vi "Disabled - Split Words from Numbers (SubVI).vi"(7 "Force Reload":bool, 9 "Input Array":string[](array[string]), 11 "File Name":string="Constants.pi") -> (2 "Numeric Array":dbl[](array[numeric]), 3 "Header Array":string[](array[string]))   [LabVIEW 2019]
doc: "Takes a file of the format:\n Line 1: Description\n Line 2: Value\n Line 3: Description\n Line 4: Value\nAnd splits it into a string array of descriptions and a numeric array of constants."
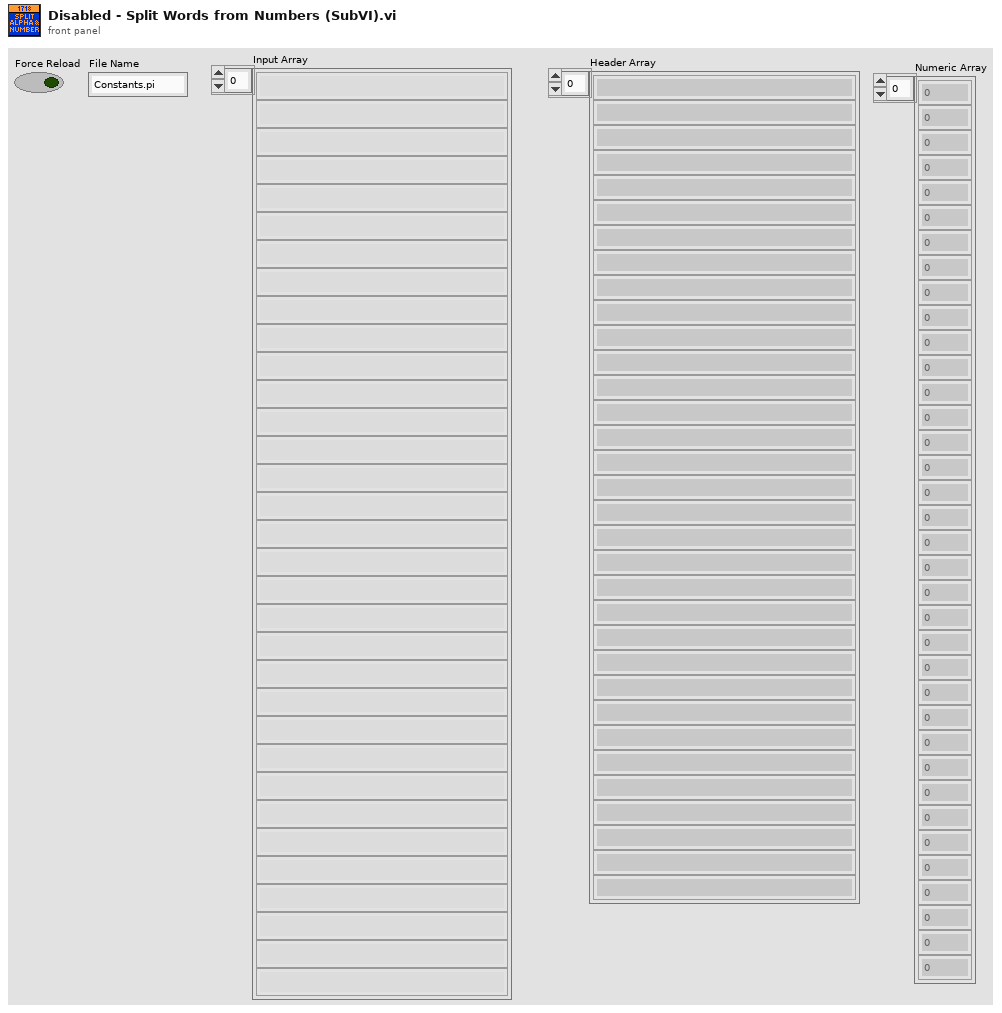
[diagram p1: front panel]
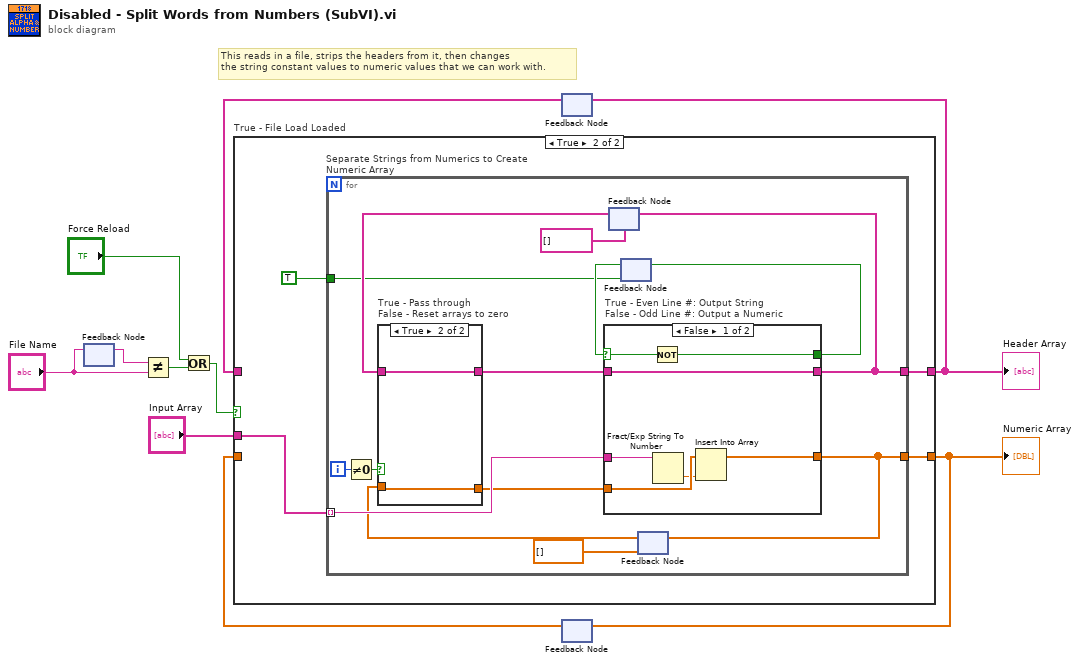
[diagram p0: block diagram]
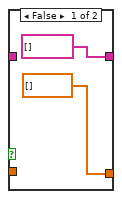
[diagram p3: hidden frame]
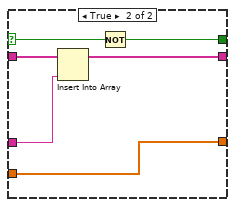
[diagram p4: hidden frame]
diagram:
  # "This reads in a file, strips the headers from it, then changes\nthe string constant values to numeric values that we can work with."
  n1 = feedback-in #1("File Name") -> ()
  n2 = feedback #1() -> (w4:string)  [unwired: 1 in]
  n3 = Not Equal?(x=w4, y="File Name") -> (x != y?=w3:bool)
  n4 = Or(x="Force Reload", y=w3) -> (x .or. y?=w1:bool)
  n5 = feedback #2() -> (w6:string[])  [unwired: 1 in]
  n6 = feedback #3() -> (w7:dbl[])  [unwired: 1 in]
  n7 = case "True - File Load Loaded" shown="True" w1 {
    tunnel: [w12 w16] -> w8
    tunnel: [w11 w15] -> w9
    tunnel: "Input Array" -> [_ w13]
    tunnel: w7 -> [w12 _]
    tunnel: w6 -> [w11 _]
    frame False {
    }
    frame True {
      n8 = for "Separate Strings from Numerics to Create Numeric Array" {
        tunnel: w13 -> [w28] mode=indexing
        tunnel: TRUE -> [w19]
        tunnel: [w25] -> w15
        tunnel: [w24] -> w16
        i -> [w17]
        n9 = Not Equal To 0?(x=w17) -> (x != 0?=w18:bool)
        n10 = feedback #4(string[] [] ("array")) -> (w23:string[])
        n11 = feedback #5(w19) -> (w29:bool)
        n12 = feedback #6(dbl[] [] ("array")) -> (w22:dbl[])
        n13 = case "True - Pass through\nFalse - Reset arrays to zero" shown="True" w18 {
          tunnel: w23 -> [_ w34]
          tunnel: w22 -> [_ w33]
          tunnel: [string[] [] ("array") w34] -> w21
          tunnel: [dbl[] [] ("array") w33] -> w20
          frame False {
          }
          frame True {
          }
        }
        n14 = case "True - Even Line #: Output String\nFalse - Odd Line #: Output a Numeric" shown="False" w29 {
          selector: w29 -> [w41 w47]
          tunnel: [w40 w46] -> w30
          tunnel: w28 -> [w37 w43]
          tunnel: w20 -> [w39 w45]
          tunnel: [w38 w45] -> w24
          tunnel: w21 -> [w35 w44]
          tunnel: [w35 w42] -> w25
          frame False {
            n15 = Not(x=w41) -> (.not. x?=w40:bool)
            n16 = Fract/Exp String To Number(string=w37) -> (number=w36:dbl)  [unwired: 3 in, 1 out]
            n17 = Insert Into Array(array=w39, new element=w36) -> (w38:dbl[])  [unwired: 1 in]
          }
          frame True {
            n18 = Insert Into Array(array=w44, new element=w43) -> (w42:string[])  [unwired: 1 in]
            n19 = Not(x=w47) -> (.not. x?=w46:bool)
          }
        }
        n20 = feedback-in #4(w25) -> ()
        n21 = feedback-in #5(w30) -> ()
        n22 = feedback-in #6(w24) -> ()
      }
    }
  }
  "Numeric Array" <- w8
  "Header Array" <- w9
  n23 = feedback-in #2(w9) -> ()
  n24 = feedback-in #3(w8) -> ()
